vi "chiller.vi"(8 "error out":errorcluster, 10 "y":bool, 11 "VISA resource name out":refnum<visa-resource-name>) -> (0 "error out 2":errorcluster, 2 "x .or. y?":bool, 3 "VISA resource name out 2":refnum<visa-resource-name>)   [LabVIEW 2019]
panel:
  out "COMBO COMMAND":string
  in  "write":bool
  out "string from combo":string
  in  "Temperature":dbl
  in  "Combo Box":string(combo)
  in  "delay before read (ms)":u32=500
  in  "read":bool=TRUE
  out "bytes read":u32
  out "chiller readout":string
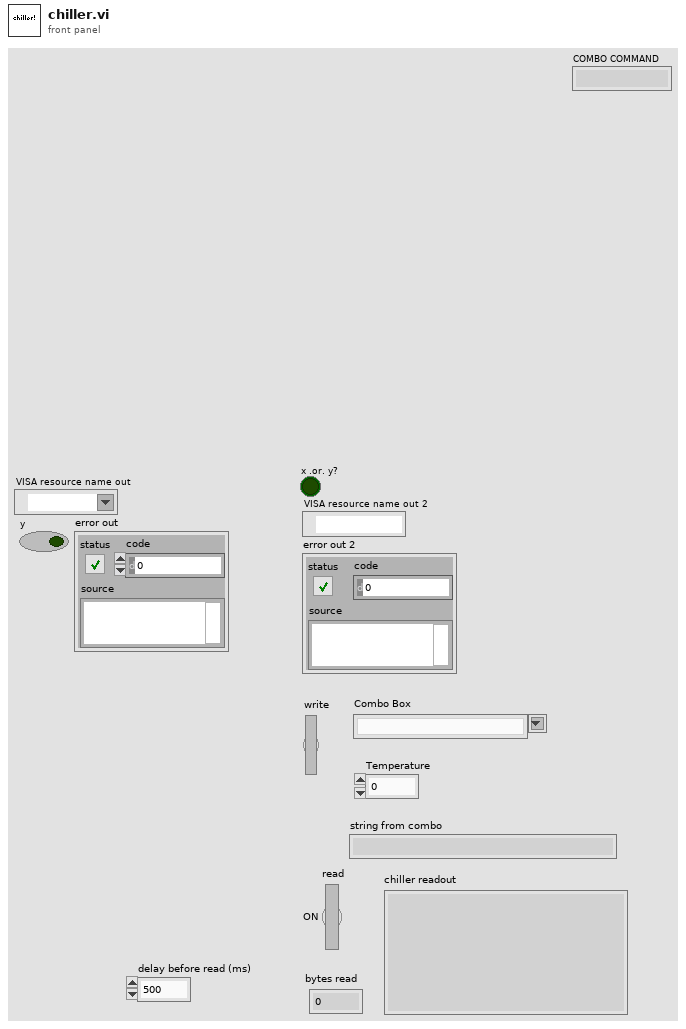
[diagram p1: front panel]
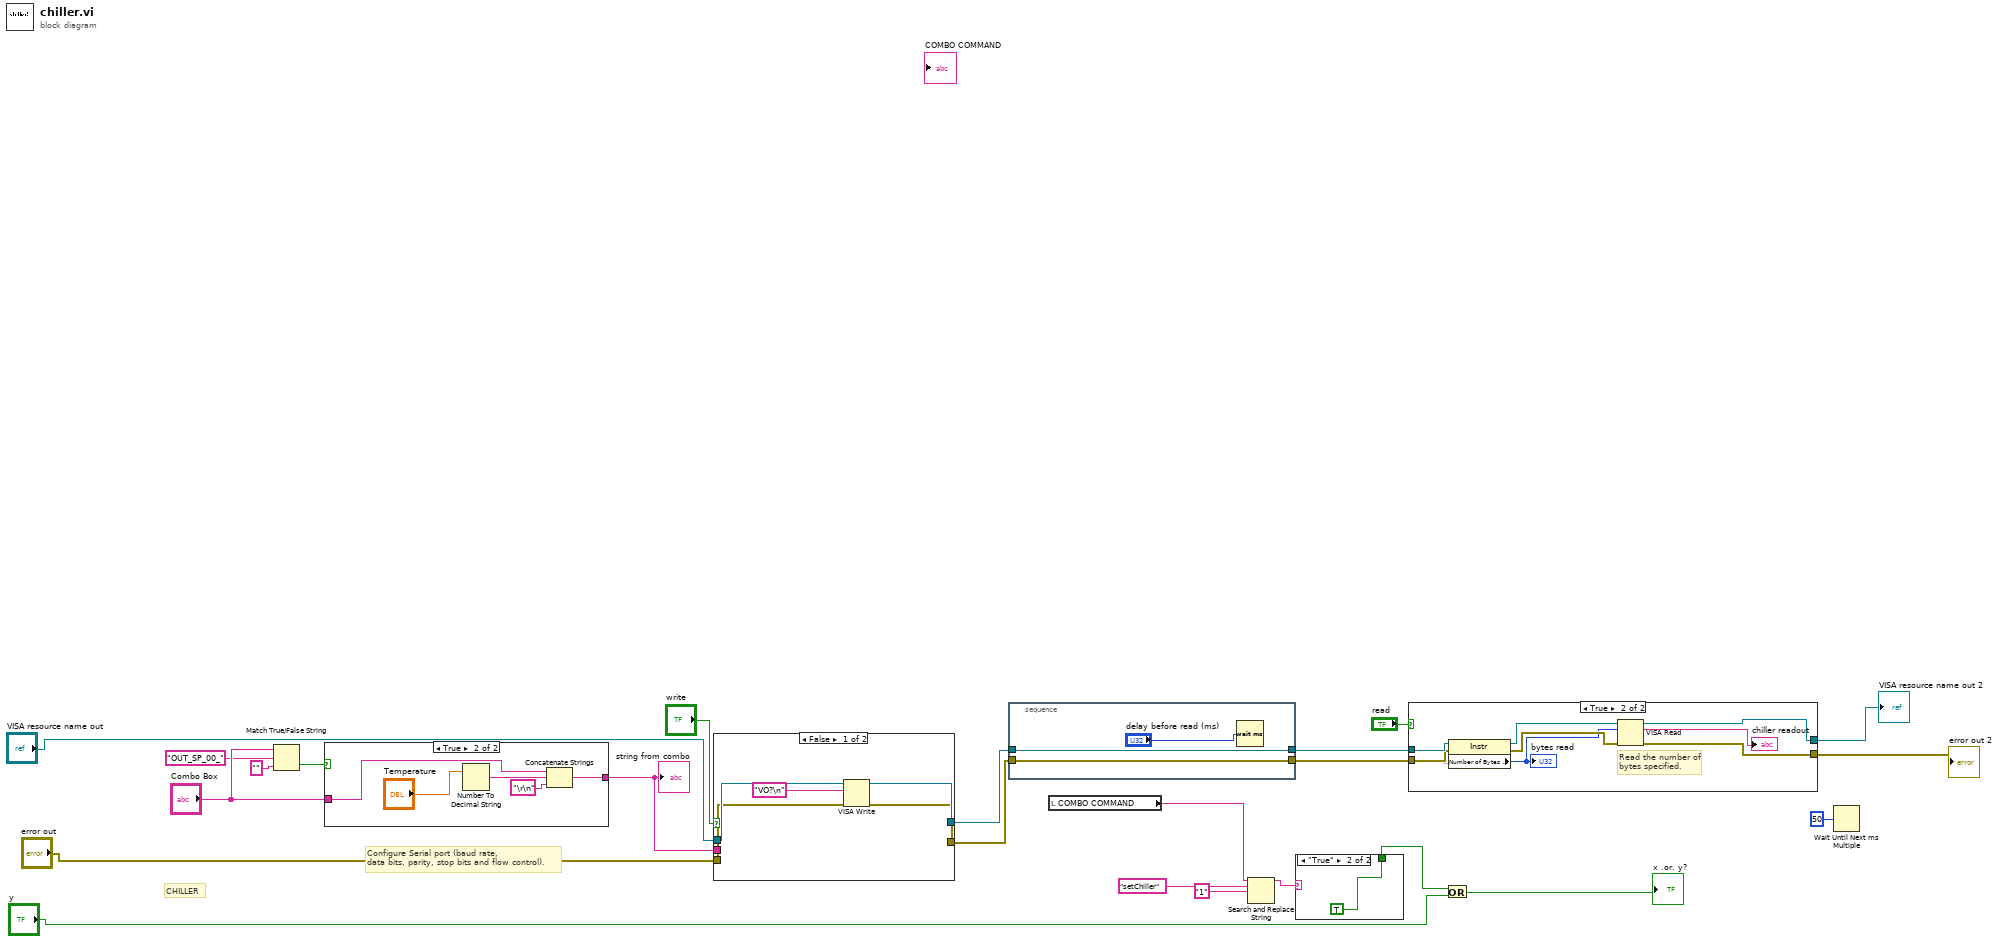
[diagram p0: block diagram]
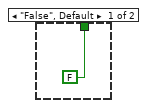
[diagram p2: hidden frame]
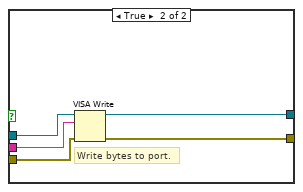
[diagram p4: hidden frame]
diagram:
  # "CHILLER"
  # "Configure Serial port (baud rate,\ndata bits, parity, stop bits and flow control)."
  n1 = Match True/False String(2:"" ("false string"), 3:"OUT_SP_00_" ("format string"), 4:"Combo Box") -> (0:w14:bool)  [unwired: 1 out]
  n2 = case shown="True" w14 {
    tunnel: [w24 w27] -> w11
    tunnel: "Combo Box" -> [w24 w26]
    frame False {
    }
    frame True {
      n3 = Number To Decimal String(number="Temperature") -> (decimal integer string=w29:string)  [unwired: 1 in]
      n4 = Concatenate Strings(w26, w29, "\r\n" ("string")) -> (w27:string)
    }
  }
  "string from combo" <- w11
  n5 = case shown="False" "write" {
    tunnel: [w30 w39] -> w20
    tunnel: "VISA resource name out" -> [w34 w38]
    tunnel: "error out" -> [w33 w37]
    tunnel: [w31 w36] -> w18
    tunnel: w11 -> [_ w35]
    frame False {
      n6 = VISA Write(VISA resource name=w34, write buffer="VO?\n", error in (no error)=w33) -> (VISA resource name out=w31:refnum<visa-resource-name>, error out=w30:errorcluster)  [unwired: 1 out]
    }
    frame True {
      # "Write bytes to port."
      n7 = VISA Write(VISA resource name=w38, write buffer=w35, error in (no error)=w37) -> (VISA resource name out=w36:refnum<visa-resource-name>, error out=w39:errorcluster)  [unwired: 1 out]
    }
  }
  n8 = stacked-sequence {
    tunnel: w20 -> [w42]
    tunnel: [w42] -> w19
    tunnel: w18 -> [w41]
    tunnel: [w41] -> w17
    frame #0 {
      n9 = Wait (ms)(milliseconds to wait="delay before read (ms)") -> ()  [unwired: 1 out]
    }
  }
  n10 = local read "COMBO COMMAND"() -> (w4:string)
  n11 = Search and Replace String(input string=w4, search string="setChiller", replace string="1" ("replace string (\"\")")) -> (result string=w9:string)  [unwired: 5 in, 3 out]
  n12 = case shown="\"True\"" w9 {
    tunnel: [FALSE TRUE] -> w6
    frame "False", Default {
    }
    frame "True" {
    }
  }
  n13 = case shown="True" "read" {
    tunnel: w19 -> [w46 w50]
    tunnel: [w46 w54] -> w22
    tunnel: [w45 w53] -> w21
    tunnel: w17 -> [w45 w52]
    frame False {
    }
    frame True {
      # "Read the number of bytes specified."
      n14 = property class="Instr"(reference=w52, error in=w50) -> (reference out=w51:refnum<visa-resource-name>, error out=w49:errorcluster, "Serial Settings:Number of Bytes at Serial Port"=w48:u32)
      "bytes read" <- w48
      n15 = VISA Read(VISA resource name=w51, byte count=w48, error in (no error)=w49) -> (VISA resource name out=w53:refnum<visa-resource-name>, read buffer=→"chiller readout":string, error out=w54:errorcluster)  [unwired: 1 out]
    }
  }
  "VISA resource name out 2" <- w21
  "error out 2" <- w22
  n16 = Or(x=w6, y="y") -> (x .or. y?=→"x .or. y?":bool)
  n17 = Wait Until Next ms Multiple(millisecond multiple=u32 50) -> ()  [unwired: 1 out]
